vi "PrototypeUI.vi"() -> ()   [LabVIEW 2017, in "Client.lvlib"]
uses:
  Client.lvlib
  CommunicationsFrameWork/TypeDefs/InternalData.ctl
  CommunicationsFrameWork/CommsFrameWork.lvlib
panel:
  in  "Support Availability 3":u32(colorbox)=3079936
  in  "Expand":bool
  in  "Support Availability 2":u32(colorbox)=3079936
  in  "Team Details":string(tree)
  in  "Phone Availability":u32(colorbox)=3079936
  in  "Suport Availability":u32(colorbox)=3079936
  in  "SRs Tab":enum32{"Unassigned", "Assigned", "Debug"}(tab)
  out "Total Unassigned":u32
  out "Prio 4 Unassigned":u32
  out "Prio 3 Unassigned":u32
  out "Prio 2 Unassigned":u32
  out "Prio 1 Unassigned":u32
  in  "Unassigned Sorted SRs":string(tree)
  in  "Assigned Sorted SRs":string(tree)
  in  "Update Connection Settings":bool
  in  "InternalData":T1={"Connection Data"={"IP"="127.0.0.1", "Port"="8001", "ClientName"="Testing"}}
  in  "Reset SR Lists":bool
  out "INI Content":string
  out "INI Path":path
  in  "Read INI":bool
  out "Last Error Detected":errorcluster
  in  "Text":string="Manual Log Entry"
  in  "Type":string="Event"
  in  "Generate Log Entry":bool
  in  "Injected Error":errorcluster
  in  "Generate Error":bool
  # "Phone Support Coverage"
  # "Suport Availability"
  # "9"
  # "Unassigned SRs:"
  # "Total:"
  # "Priority 2"
  # "Priority 1"
  # "Priority 3"
  # "Priority 4"
  # "Manual Controls"
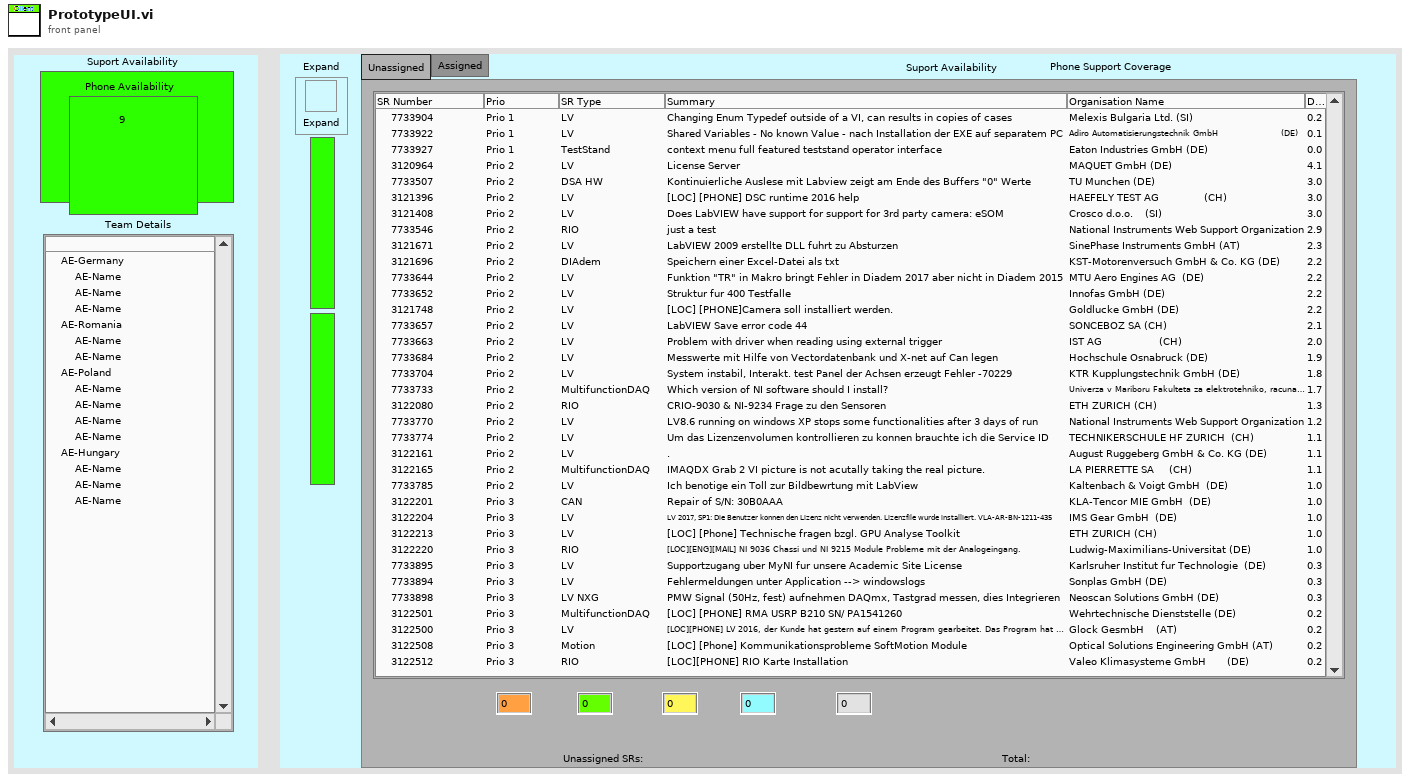
[diagram p1: front panel]
types:
  T1 = typedef "Client.lvlib/CommsFrameWork.lvlib/InternalData.ctl" = cluster{"Connection Data":cluster{"IP":string, "Port":string, "ClientName":string}}
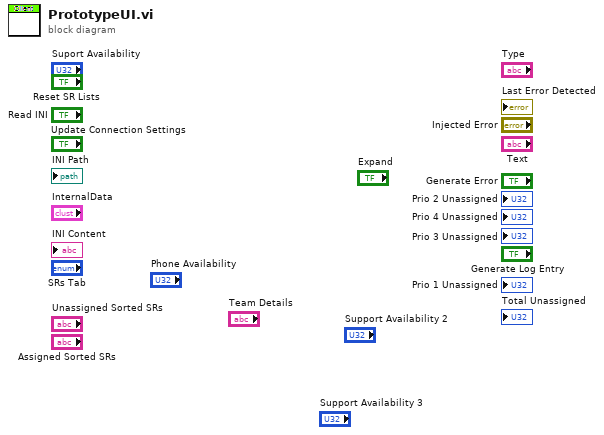
[diagram p0: block diagram]
diagram:
